vi "settings.vi"(6 "refresh":bool, 8 "Update":bool, 11 "New Values":string[](array[string])) -> (0 "Values":string[](array[string]), 3 "Keys":string[](array[string]), 4 "Refresh?":bool)   [LabVIEW 2015]
uses:
  <vilib>/Rock Robotics/Network Tables/NT Read Boolean.vi
  <vilib>/Rock Robotics/Network Tables/NT Write Boolean.vi
  <vilib>/Rock Robotics/Network Tables/NT Write String.vi
  <vilib>/Rock Robotics/Network Tables/NT Read Number.vi
  <vilib>/Rock Robotics/Network Tables/NT Read String.vi
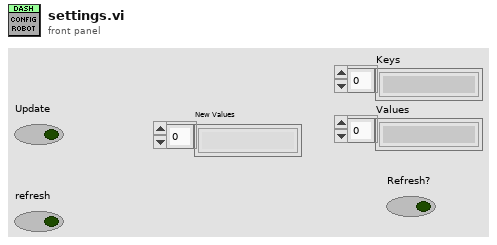
[diagram p1: front panel]
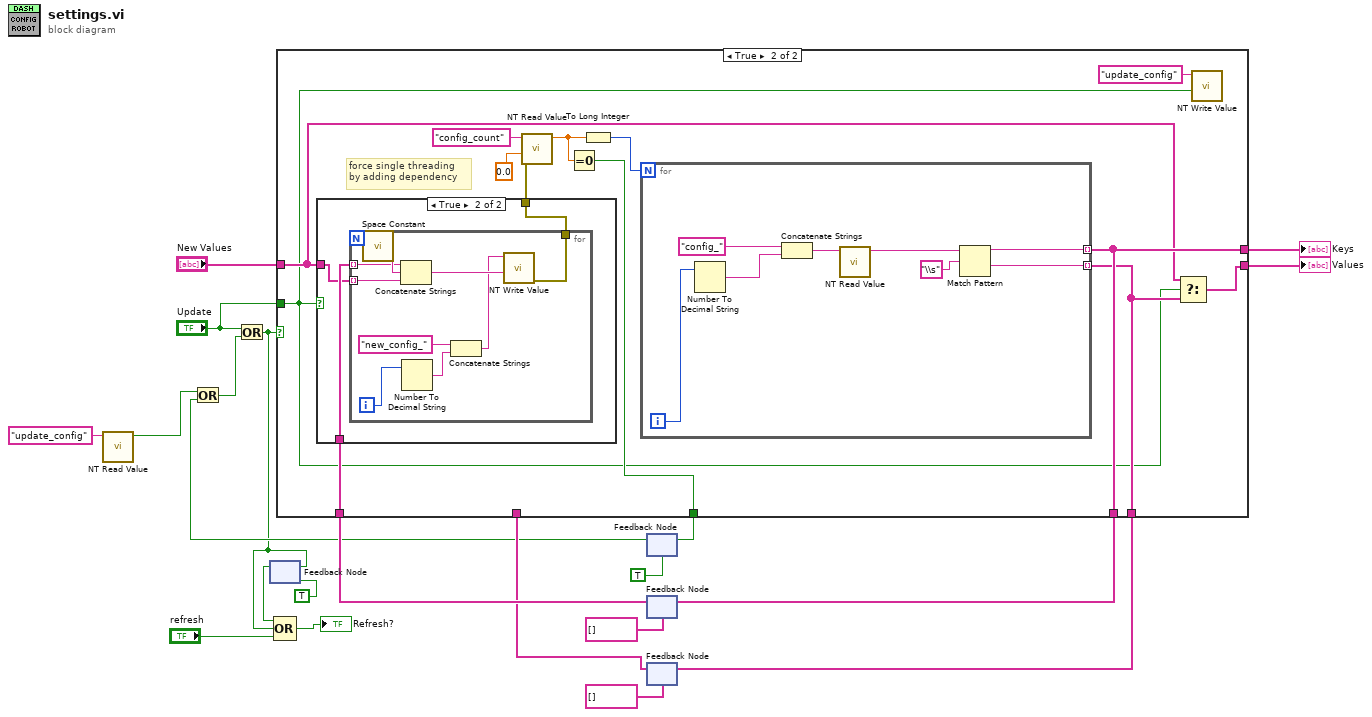
[diagram p0: block diagram]
diagram:
  n1 = call-poly <vilib>:"NT Read Value.vi"("Name"="update_config") -> ("Boolean"=w6:bool)  [unwired: 9 in, 1 out]
  n2 = feedback #1(TRUE) -> (w5:bool)
  n3 = feedback #2(TRUE) -> (w8:bool)
  n4 = Or(x=w6, y=w8) -> (x .or. y?=w7:bool)
  n5 = Or(x="Update", y=w7) -> (x .or. y?=w4:bool)
  n6 = feedback-in #1(w4) -> ()
  n7 = Compound Arithmetic op=OR(w5, w4, "refresh") -> (→"Refresh?":bool)
  n8 = feedback #3(string[] []) -> (w18:string[])
  n9 = feedback #4(string[] []) -> (w11:string[])
  n10 = case shown="True" w4 {
    selector: w4 -> [w24 _]
    tunnel: [w24 w30] -> w10
    tunnel: "New Values" -> [_ w26]
    tunnel: [w22 w33] -> w19
    tunnel: w18 -> [w22 w35]
    tunnel: "Update" -> [_ w25]
    tunnel: [w22 w33] -> w15
    tunnel: [w23 w27] -> w14
    tunnel: [w23 w28] -> w12
    tunnel: w11 -> [w23 _]
    frame False {
    }
    frame True {
      # "force single threading\nby adding dependency"
      n11 = case shown="True" w25 {
        tunnel: w35 -> [_ w40]
        tunnel: w26 -> [_ w39]
        tunnel: [_ w38] -> w34
        frame False {
        }
        frame True {
          n12 = for {
            tunnel: w40 -> [w42] mode=indexing
            tunnel: w39 -> [w41] mode=indexing
            tunnel: [w43] -> w38
            i -> [w45]
            n13 = call <vilib>:"Space Constant.vi"() -> ("String"=w49:string)
            n14 = Concatenate Strings(w42, w49, w41) -> (w48:string)
            n15 = Number To Decimal String(number=w45) -> (decimal integer string=w47:string)  [unwired: 1 in]
            n16 = Concatenate Strings("new_config_" ("Name"), w47) -> (w44:string)
            n17 = call-poly <vilib>:"NT Write Value.vi"("String"=w48, "Name"=w44) -> ("error out"=w43:errorcluster)  [unwired: 9 in]
          }
        }
      }
      n18 = call-poly <vilib>:"NT Read Value.vi"("error in"=w34, "Default Value"=0.0, "Name"="config_count") -> ("Numeric"=w31:dbl)  [unwired: 7 in, 1 out]
      n19 = Equal To 0?(x=w31) -> (x = 0?=w30:bool)
      n20 = To Long Integer(number=w31) -> (32bit integer=w36:i32)
      n21 = for {
        N: w36 -> [_]
        tunnel: [w51] -> w33 mode=indexing
        tunnel: [w50] -> w28 mode=indexing
        i -> [w56]
        n22 = Number To Decimal String(number=w56) -> (decimal integer string=w55:string)  [unwired: 1 in]
        n23 = Concatenate Strings("config_" ("Name"), w55) -> (w54:string)
        n24 = call-poly <vilib>:"NT Read Value.vi"("Name"=w54) -> ("String"=w53:string)  [unwired: 9 in, 1 out]
        n25 = Match Pattern(string=w53, regular expression="\\s") -> (before substring=w51:string, after substring=w50:string)  [unwired: 1 in, 2 out]
      }
      n26 = Select(t=w26, s=w25, f=w28) -> (s? t:f=w27:string[])
      n27 = call-poly <vilib>:"NT Write Value.vi"("Boolean"=w25, "Name"="update_config") -> ()  [unwired: 9 in, 1 out]
    }
  }
  "Keys" <- w15
  "Values" <- w14
  n28 = feedback-in #2(w10) -> ()
  n29 = feedback-in #3(w19) -> ()
  n30 = feedback-in #4(w12) -> ()
